vi "Create.vi"(8 "error in (no error)":errorcluster, 10 "Panel":refnum<k24>(container), 11 "LV MDI in":refnum<class "LV MDI.lvclass">) -> (0 "error out":errorcluster, 3 "LV MDI out":refnum<class "LV MDI.lvclass">)   [LabVIEW 2016, in "LV MDI.lvclass"]
doc: "Create reference for MDI Panel."
uses:
  LV MDI.lvclass
  System.Windows.Forms
  LV MDI.lvclass/LV MDI.ctl
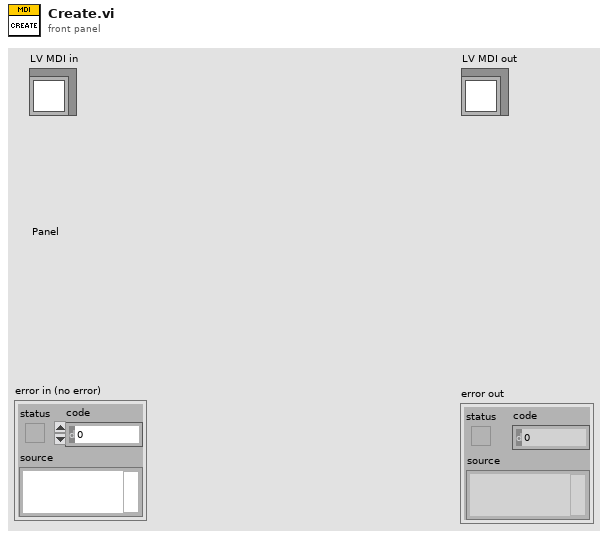
[diagram p1: front panel]
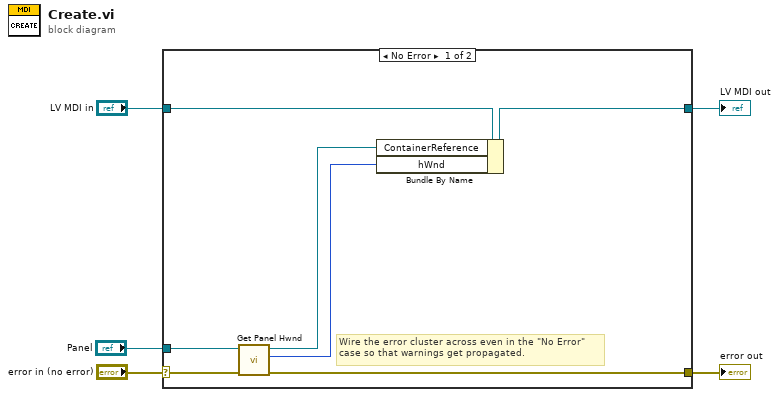
[diagram p0: block diagram]
diagram:
  n1 = case shown="No Error" "error in (no error)" {
    selector: "error in (no error)" -> [w11 w14]
    tunnel: [w10 w14] -> w4
    tunnel: [w8 w13] -> w2
    tunnel: "LV MDI in" -> [w9 w13]
    tunnel: "Panel" -> [w12 _]
    frame No Error {
      # "Wire the error cluster across even in the \"No Error\"\ncase so that warnings get propagated."
      n2 = call "Get Panel Hwnd.vi"("error in (no error)"=w11, "Panel"=w12) -> ("error out"=w10:errorcluster, "HWND"=w6:u64, "Container reference out"=w7:refnum<k24>)  [unwired: 7 in]
      n3 = Bundle By Name(cluster=w9, "ContainerReference"=w7, "hWnd"=w6) -> (w8:refnum<class "LV MDI.lvclass">)
    }
    frame Error {
    }
  }
  "error out" <- w4
  "LV MDI out" <- w2
